vi "CheckTemperature.vi"(8 "error in (no error)":errorcluster, 11 "temperature in":i32) -> (0 "error out":errorcluster)   [LabVIEW 2009]
uses:
  Utilities/controls/ctlSeqFNs_Andor_temp.ctl
  Variables/GlobalCameraHandle.vi
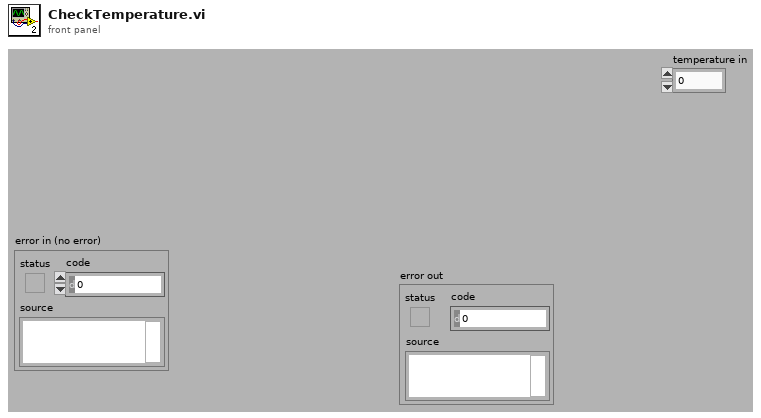
[diagram p1: front panel]
types:
  T1 = typedef "ctlSeqFNs_Andor_temp.ctl" = enum16{"Temperature  FALSE", "Temperature OK"}
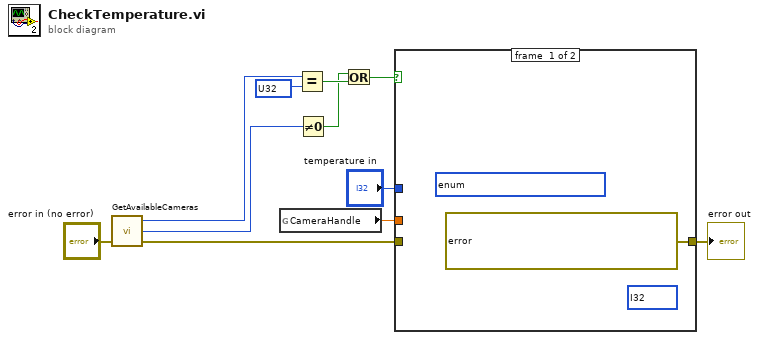
[diagram p0: block diagram]
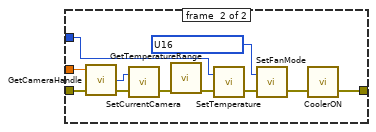
[diagram p2: hidden frame]
diagram:
  n1 = call "GetAvailableCameras.vi"("error in (no error)"="error in (no error)") -> ("error out"=w5:errorcluster, "totalCameras"=w4:i32, "DLL error code"=w11:u32)  [unwired: 2 in]
  n2 = global read "GlobalCameraHandle.vi" "CameraHandle"() -> (w1:dbl)
  n3 = Equal?(x=w11, y=u32 ?) -> (x = y?=w9:bool)
  n4 = Not Equal To 0?(x=w4) -> (x != 0?=w2:bool)
  n5 = Or(x=w2, y=w9) -> (x .or. y?=w7:bool)
  n6 = case shown="True" w7 {
    tunnel: [errorcluster ? ("error out") w23] -> w6
    tunnel: w5 -> [_ w22]
    tunnel: "temperature in" -> [_ w21]
    tunnel: w1 -> [_ w13]
    frame #0 {
      (unwired) i32[] ?
      (unwired) T1[] ? items=["Temperature  FALSE", "Temperature OK"]
    }
    frame #1 {
      w18 = u16 ? items=["Fan Mode Full", "Fan Mode Half", "Fan Mode Low"] ("Ring")
      n7 = call "GetCameraHandle.vi"("error in (no error)"=w22, "cameraIndex"=w13) -> ("error out"=w17:errorcluster, "cameraHandle"=w16:i32)  [unwired: 1 in, 1 out]
      n8 = call "SetCurrentCamera.vi"("error in (no error)"=w17, "cameraHandle"=w16) -> ("error out"=w15:errorcluster)  [unwired: 1 out]
      n9 = call "GetTemperatureRange.vi"("error in (no error)"=w15) -> ("error out"=w20:errorcluster)  [unwired: 3 in, 3 out]
      n10 = call "SetTemperature.vi"("error in (no error)"=w20, "temperature"=w21) -> ("error out"=w19:errorcluster)  [unwired: 1 out]
      n11 = call "SetFanMode.vi"("error in (no error)"=w19, "mode"=w18) -> ("error out"=w14:errorcluster)  [unwired: 1 out]
      n12 = call "CoolerON.vi"("error in (no error)"=w14) -> ("error out"=w23:errorcluster)  [unwired: 1 in, 1 out]
    }
  }
  "error out" <- w6
